vi "Read.vi"(8 "error in (no error)":errorcluster, 10 "Timeout(10000 ms)":u32=10000, 11 "VISA resource name":refnum<visa-resource-name>) -> (0 "error out":errorcluster, 2 "Measurement":T1 {"Measurement" format="%.6e"}, 3 "VISA resource name out":refnum<visa-resource-name>)   [LabVIEW 2016, in "Keithley 6517.lvlib"]
doc: "Reads the measurement from the instrument."
uses:
  <instrlib>/Keithley 6517/Keithley 6517.lvlib
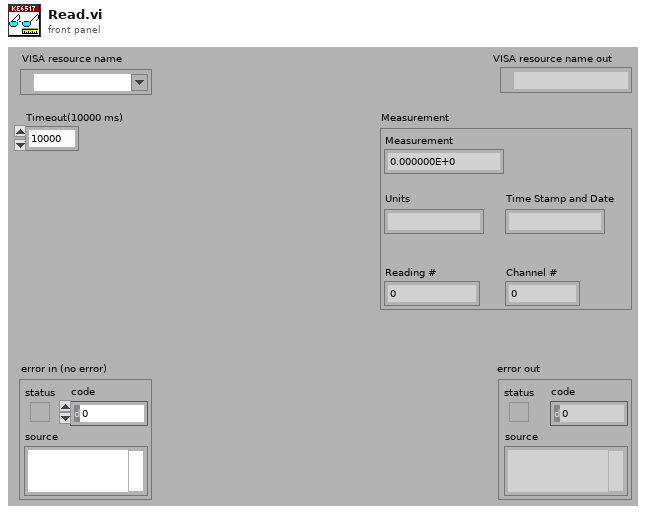
[diagram p1: front panel]
types:
  T1 = cluster{"Measurement":dbl, "Units":string, "Time Stamp and Date":string, "Reading #":dbl, "Channel #":dbl}
  T2 = typedef "Keithley 6517.lvlib/Extended User Data.ctl" = cluster{"Instrument Model":i32}
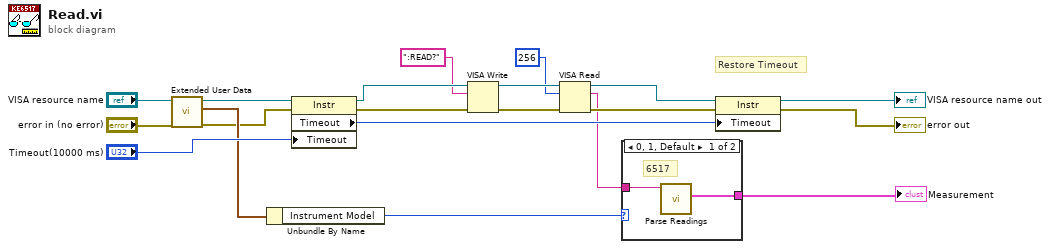
[diagram p0: block diagram]
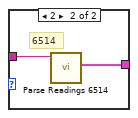
[diagram p2: hidden frame]
diagram:
  # "Restore Timeout"
  n1 = call <instrlib>:"Extended User Data.vi"("error in (no error)"="error in (no error)", "VISA resource name"="VISA resource name") -> ("error out"=w1:errorcluster, "User Data Out"=w6:T2, "VISA resource name out"=w2:refnum<visa-resource-name>)  [unwired: 7 in]
  n2 = Unbundle By Name(w6) -> ("Instrument Model"=w5:i32)
  n3 = property class="Instr"(reference=w2, error in=w1, "Timeout"="Timeout(10000 ms)") -> (reference out=w19:refnum<visa-resource-name>, error out=w20:errorcluster, "Timeout"=w11:u32)
  n4 = VISA Write(VISA resource name=w19, write buffer=":READ?", error in (no error)=w20) -> (VISA resource name out=w17:refnum<visa-resource-name>, error out=w16:errorcluster)  [unwired: 1 out]
  n5 = VISA Read(VISA resource name=w17, byte count=u32 256, error in (no error)=w16) -> (VISA resource name out=w10:refnum<visa-resource-name>, read buffer=w4:string, error out=w9:errorcluster)  [unwired: 1 out]
  n6 = case shown="0, 1, Default" w5 {
    tunnel: w4 -> [w22 w24]
    tunnel: [w21 w23] -> w3
    frame 0, 1, Default {
      # "6517"
      n7 = call <instrlib>:"Parse Readings.vi"("Readings"=w22) -> ("Measurement"=w21:T1)  [unwired: 9 in, 1 out]
    }
    frame 2 {
      # "6514"
      n8 = call <instrlib>:"Parse Readings 6514.vi"("Readings"=w24) -> ("Measurement"=w23:T1)  [unwired: 9 in, 1 out]
    }
  }
  "Measurement" <- w3
  n9 = property class="Instr"(reference=w10, error in=w9, "Timeout"=w11) -> (reference out=→"VISA resource name out":refnum<visa-resource-name>, error out=→"error out":errorcluster)
